vi "Utility Format Head Type.vi"(8 "error in (no error)":errorcluster, 11 "Head Type":i32) -> (0 "error out":errorcluster, 3 "Formatted Head Type":string)   [LabVIEW 2020, in "ChromTech Series III Pump.lvlib"]
uses:
  <instrlib>/RxnRover/ChromtechSeriesIIIDriver/ChromTech Series III Pump.lvlib
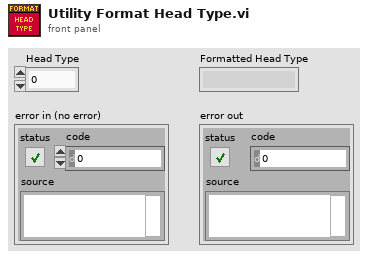
[diagram p1: front panel]
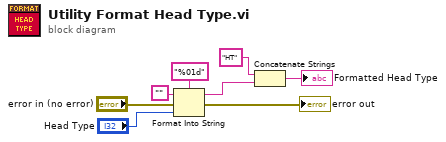
[diagram p0: block diagram]
diagram:
  n1 = Format Into String(format string="%01d", initial string="", error in="error in (no error)", "Head Type") -> (resulting string=w4:string, error out=→"error out":errorcluster)
  n2 = Concatenate Strings("HT", w4) -> (→"Formatted Head Type":string)
